vi "Ramp to Set.vi"(6 "Axis":T1, 8 "error in (no error)":errorcluster, 11 "Instrument.VRM in":refnum<class "Instrument.OxfordVRM.lvclass">) -> (0 "error out":errorcluster, 2 "Response":string, 3 "Instrument.VRM out":refnum<class "Instrument.OxfordVRM.lvclass">)   [LabVIEW 2016, in "Instrument.OxfordVRM.lvclass"]
uses:
  Instrument.OxfordVRM.lvclass
  <userlib>/LevyLab/Levylab Instruments/Instrument Types/Cryostat/Typedefs/VRM Magnet Axis--Enum.ctl
  <instrlib>/Mercury iXX/Public/Libraries/Magnet/Controls/PSU Actions.ctl
  Typedefs/Instrument.VRM.Commands-enum.ctl
  Typedefs/VRM Action-Axis--Cluster.ctl
  <instrlib>/Mercury iXX/Public/Libraries/Magnet.lvlib
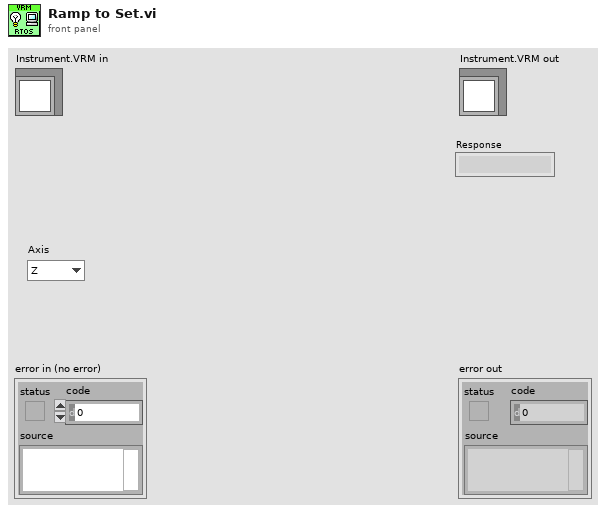
[diagram p1: front panel]
types:
  T1 = typedef "Instrument.OxfordVRM.lvclass/VRM Magnet Axis--Enum.ctl" = enum16{"Z", "X", "Y", "ALL"}
  T2 = typedef "Instrument.OxfordVRM.lvclass/VRM Action-Axis--Cluster.ctl" = cluster{"PSU Act Stat":T3, "Axis":T1}
  T3 = typedef "Mercury iXX.lvlib/Magnet.lvlib/PSU Actions.ctl" = string
  T4 = typedef "Instrument.OxfordVRM.lvclass/Instrument.VRM.Commands-enum.ctl" = enum16{"setAction", "setTarget", "setMagnetField", "getStatus", "getTarget", "getMagnetField"}
  T5 = cluster{"Holding":bool, "Ramp to Setpoint":bool, "Ramp to Zero":bool, "Clamp":bool}
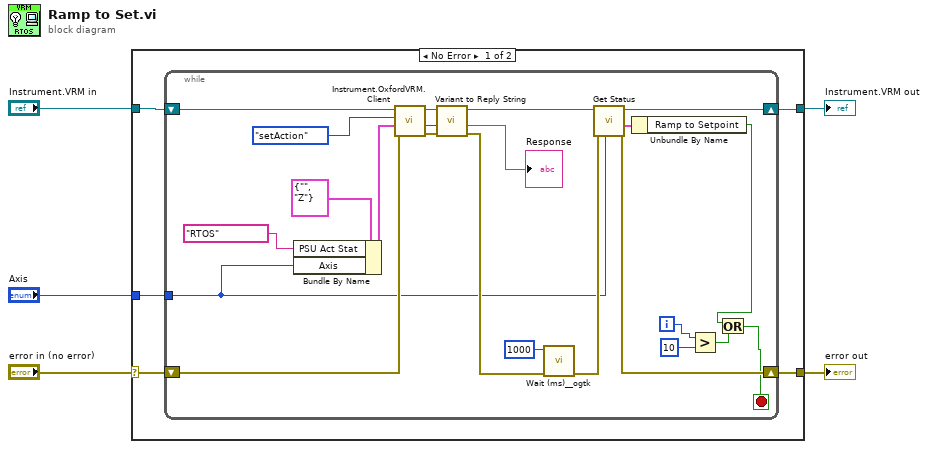
[diagram p0: block diagram]
diagram:
  n1 = case shown="No Error" "error in (no error)" {
    selector: "error in (no error)" -> [w9 w35]
    tunnel: [w8 w35] -> w4
    tunnel: [w7 w34] -> w2
    tunnel: "Instrument.VRM in" -> [w10 w34]
    tunnel: "Axis" -> [w6 _]
    frame No Error {
      n2 = while {
        shift-right: [w28] -> w7
        shift-left: w10 -> [w27]
        shift-right: [w29] -> w8
        shift-left: w9 -> [w33]
        tunnel: w6 -> [w14]
        i -> [w11]
        stop <- w23 stop-if-true
        n3 = Bundle By Name(cluster=T2 {"PSU Act Stat"="", "Axis"=enum."Z"} ("Action"), "PSU Act Stat"=T3 "RTOS", "Axis"=w14) -> (w13:T2)
        n4 = call "Instrument.OxfordVRM.Client.vi"("error in (no error)"=w33, "Data"=w13, "Commands"=Instrument.VRM.Commands-enum."setAction", "Instrument.VRM in"=w27) -> ("error out"=w20:errorcluster, "Data out"=w22:variant, "Instrument.VRM out"=w21:refnum<class "Instrument.OxfordVRM.lvclass">)  [unwired: 5 in]
        n5 = call "Variant to Reply String.vi"("error in (no error)"=w20, "Data"=w22, "Instrument.VRM in"=w21) -> ("error out"=w19:errorcluster, "Reply"=→"Response":string, "Instrument.VRM out"=w18:refnum<class "Instrument.OxfordVRM.lvclass">)  [unwired: 6 in]
        n6 = call <userlib>:"Wait (ms)__ogtk.vi"("error in (no error)"=w19, "milliseconds to wait"=u32 1000) -> ("error out"=w30:errorcluster)  [unwired: 8 in, 1 out]
        n7 = call "Get Status.vi"("Axis"=w14, "error in (no error)"=w30, "Instrument.VRM in"=w18) -> ("error out"=w29:errorcluster, "Status"=w31:T5, "Instrument.VRM out"=w28:refnum<class "Instrument.OxfordVRM.lvclass">)  [unwired: 5 in, 1 out]
        n8 = Unbundle By Name(w31) -> ("Ramp to Setpoint"=w24:bool)
        n9 = Greater?(x=w11, y=10) -> (0:w25:bool)
        n10 = Or(x=w24, y=w25) -> (x .or. y?=w23:bool)
      }
    }
    frame Error {
    }
  }
  "error out" <- w4
  "Instrument.VRM out" <- w2
